vi "LogDBFeedFlash.vi"(0 "Refnum in":T1, 1 "value volume [dl]":u64, 2 "enable":bool, 3 "feeding":bool, 4 "feeding start volume":u64, 5 "feeding start time":timestamp, 6 "flashing":bool, 7 "error in":errorcluster, 8 "valve t-2 close":bool, 9 "flashing start volume":u64, 10 "valve t-1 close":bool, 11 "flashing start time":timestamp, 12 "prefix":string, 14 "Pump":bool) -> (18 "feeding":bool, 20 "Refnum out":T1, 21 "feeding start volume":u64, 22 "feeding start time":timestamp, 23 "flashing":bool, 24 "flashing start volume":u64, 25 "flashing start time":timestamp, 27 "error out":errorcluster)   [LabVIEW 2011]
uses:
  <vilib>/addons/database/Connection.llb/Conn ObjectReference.ctl
  <vilib>/addons/database/NI_Database_API.lvlib
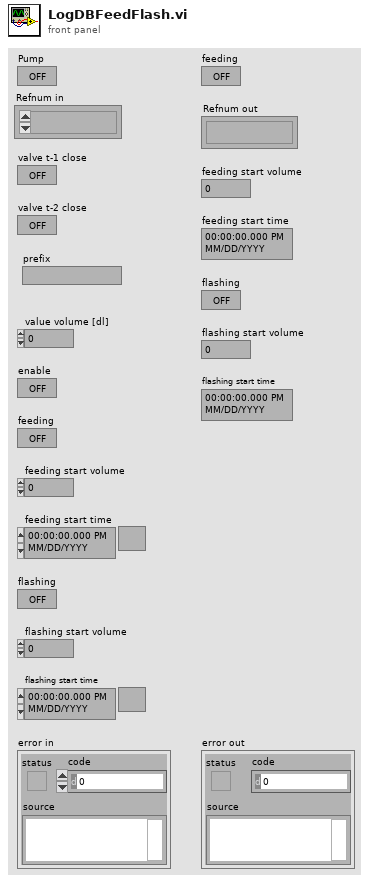
[diagram p1: front panel]
types:
  T1 = typedef "NI_Database_API.lvlib/Conn ObjectReference.ctl" = refnum<k1>
  T2 = cluster{"feeding start time":timestamp, "seconds since 1Jan1904":timestamp, u64}
  T3 = cluster{"flashing start time":timestamp, "seconds since 1Jan1904":timestamp, u64}
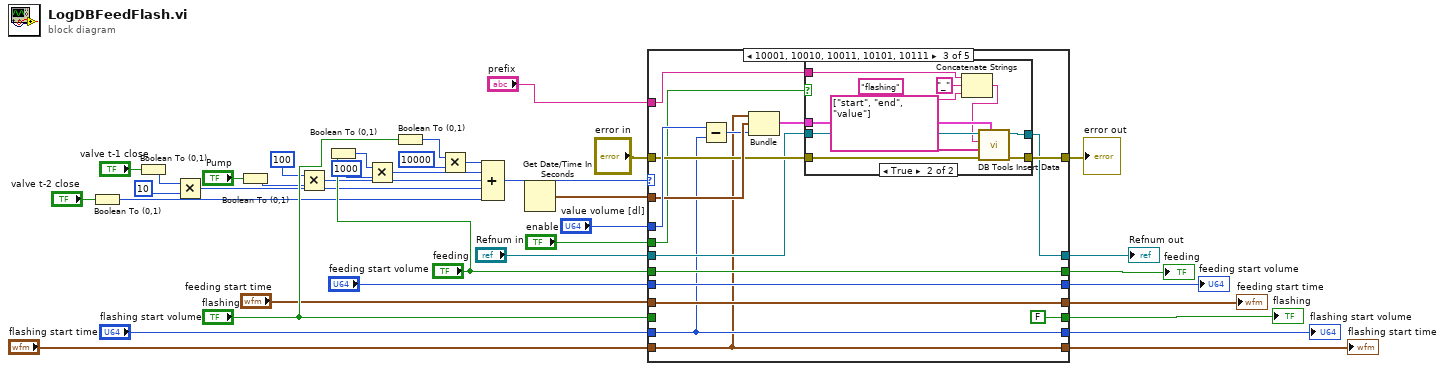
[diagram p0: block diagram]
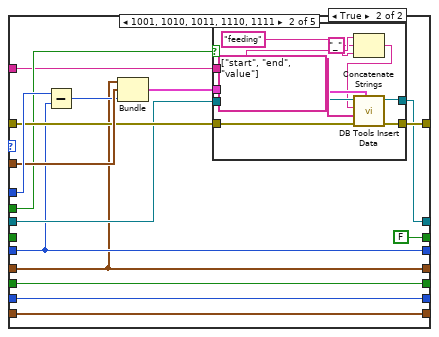
[diagram p3: hidden frame]
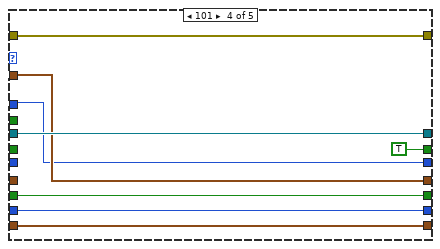
[diagram p6: hidden frame]
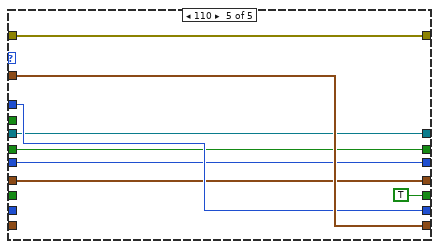
[diagram p7: hidden frame]
diagram:
  n1 = Boolean To (0,1)(Boolean="valve t-2 close") -> (0, 1=w6:i16)
  n2 = Boolean To (0,1)(Boolean="valve t-1 close") -> (0, 1=w7:i16)
  n3 = Multiply(x=w7, y=i16 10) -> (x*y=w9:i16)
  n4 = Boolean To (0,1)(Boolean="Pump") -> (0, 1=w10:i16)
  n5 = Multiply(x=i16 100, y=w10) -> (x*y=w12:i16)
  n6 = Boolean To (0,1)(Boolean="feeding") -> (0, 1=w14:i16)
  n7 = Multiply(x=w14, y=i16 1000 ("x")) -> (x*y=w15:i16)
  n8 = Boolean To (0,1)(Boolean="flashing") -> (0, 1=w21:i16)
  n9 = Multiply(x=w21, y=i16 10000 ("x")) -> (x*y=w22:i16)
  n10 = Compound Arithmetic op=ADD(w22, w15, w12, w9, w6) -> (w16:i16)
  n11 = Get Date/Time In Seconds() -> (seconds since 1Jan1904=w17:timestamp)
  n12 = case shown="10001, 10010, 10011, 10101, 10111" w16 {
    tunnel: "value volume [dl]" -> [_ w61 w89 w105 w114]
    tunnel: w17 -> [_ w60 w88 w106 w116]
    tunnel: "error in" -> [w45 w58 w86 w109 w117]
    tunnel: [w45 w57 w85 w109 w117] -> w19
    tunnel: [w44 w55 w83 w108 w113] -> w23
    tunnel: [w43 FALSE ("feeding") w77 TRUE ("feeding start") w112] -> w24
    tunnel: "enable" -> [_ w53 w81 _ _]
    tunnel: "Refnum in" -> [w44 w52 w82 w108 w113]
    tunnel: "feeding start time" -> [w39 w50 w79 _ w110]
    tunnel: "feeding start volume" -> [w38 w51 w80 _ w111]
    tunnel: [w39 w50 w79 w106 w110] -> w29
    tunnel: [w38 w51 w80 w105 w111] -> w30
    tunnel: [w42 w47 w75 w102 w116] -> w31
    tunnel: [w40 w49 FALSE ("feeding") w104 TRUE ("feeding start")] -> w32
    tunnel: [w41 w48 w76 w103 w114] -> w33
    tunnel: "flashing start volume" -> [w41 w48 w76 w103 _]
    tunnel: "flashing start time" -> [w42 w47 w75 w102 _]
    tunnel: "flashing" -> [w40 w49 _ w104 _]
    tunnel: "feeding" -> [w43 _ w77 _ w112]
    tunnel: "prefix" -> [_ w46 w74 _ _]
    frame 0, Default {
    }
    frame 1001, 1010, 1011, 1110, 1111 {
      n13 = Subtract(x=w61, y=w51) -> (x-y=w59:u64)
      n14 = Bundle("feeding start time"=w50, "seconds since 1Jan1904"=w60, w59) -> (w56:T2)  [unwired: 1 in]
      n15 = case shown="True" w53 {
        tunnel: w52 -> [w62 w72]
        tunnel: w58 -> [w63 w71]
        tunnel: [w63 w70] -> w57
        tunnel: w56 -> [_ w69]
        tunnel: [w62 w68] -> w55
        tunnel: w46 -> [_ w67]
        frame False {
        }
        frame True {
          n16 = Concatenate Strings(w67, "_" ("string"), "feeding" ("table")) -> (w64:string)
          n17 = call <vilib>:"DB Tools Insert Data.vi"("data"=w69, "error in (no error)"=w71, "columns"=string[] ["start", "end", "value"], "table"=w64, "connection reference"=w72) -> ("error out"=w70:errorcluster, "connection reference out"=w68:T1)  [unwired: 5 in]
        }
      }
    }
    frame 10001, 10010, 10011, 10101, 10111 {
      n18 = Subtract(x=w89, y=w76) -> (x-y=w87:u64)
      n19 = Bundle("flashing start time"=w75, "seconds since 1Jan1904"=w88, w87) -> (w84:T3)  [unwired: 1 in]
      n20 = case shown="True" w81 {
        tunnel: w82 -> [w90 w101]
        tunnel: w86 -> [w91 w100]
        tunnel: [w91 w99] -> w85
        tunnel: w84 -> [_ w98]
        tunnel: [w90 w97] -> w83
        tunnel: w74 -> [_ w94]
        frame False {
        }
        frame True {
          n21 = Concatenate Strings(w94, "_" ("string"), "flashing" ("table")) -> (w92:string)
          n22 = call <vilib>:"DB Tools Insert Data.vi"("data"=w98, "error in (no error)"=w100, "columns"=string[] ["start", "end", "value"], "table"=w92, "connection reference"=w101) -> ("error out"=w99:errorcluster, "connection reference out"=w97:T1)  [unwired: 5 in]
        }
      }
    }
    frame 101 {
    }
    frame 110 {
    }
  }
  "flashing start volume" <- w33
  "flashing" <- w32
  "flashing start time" <- w31
  "feeding start volume" <- w30
  "feeding start time" <- w29
  "feeding" <- w24
  "Refnum out" <- w23
  "error out" <- w19
